vi "Query Waveform Length.vi"(8 "error in (no error)":errorcluster, 10 "Memory Name (0: Edit Memory)":i32(ring) items=["Edit Memory", "Edit Memory 1", "Edit Memory 2"], 11 "VISA resource name":refnum<visa-resource-name>) -> (0 "error out":errorcluster, 2 "Query Points":i32, 3 "VISA resource name out":refnum<visa-resource-name>)   [LabVIEW 2020, in "AWG.lvlib" / "Tektronix AFG 3000 Series.lvlib"]
doc: "Gets the number of data points for the waveform created in the edit memory.\n\n<B>Note:</B>\n \nThis VI is only applicable for AFG 3KC series."
uses:
  Tektronix AFG 3000 Series.lvlib
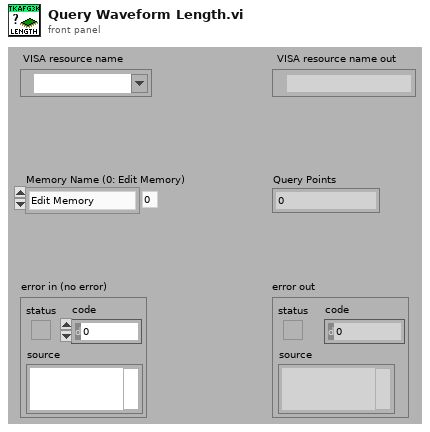
[diagram p1: front panel]
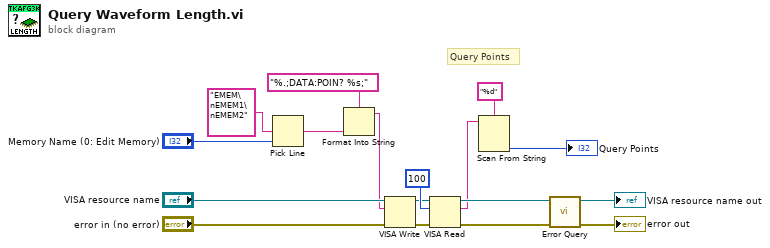
[diagram p0: block diagram]
diagram:
  # "Query Points"
  n1 = Pick Line(multi-line string="EMEM\nEMEM1\nEMEM2" ("string (\"\")"), line index="Memory Name (0: Edit Memory)") -> (output string=w15:string)  [unwired: 1 in]
  n2 = Format Into String(format string="%.;DATA:POIN? %s;", w15) -> (resulting string=w3:string)  [unwired: 2 in, 1 out]
  n3 = VISA Write(VISA resource name="VISA resource name", write buffer=w3, error in (no error)="error in (no error)") -> (VISA resource name out=w4:refnum<visa-resource-name>, error out=w5:errorcluster)  [unwired: 1 out]
  n4 = VISA Read(VISA resource name=w4, byte count=u32 100, error in (no error)=w5) -> (VISA resource name out=w11:refnum<visa-resource-name>, read buffer=w2:string, error out=w9:errorcluster)  [unwired: 1 out]
  n5 = Scan From String(format string="%d", input string=w2) -> (output 1=→"Query Points":i32)  [unwired: 3 in, 3 out]
  n6 = call "Error Query.vi"("error in (no error)"=w9, "VISA resource name"=w11) -> ("error out"=→"error out":errorcluster, "VISA resource name out"=→"VISA resource name out":refnum<visa-resource-name>)  [unwired: 6 in, 2 out]
